vi "Shooter_WinchNoPID.vi"(6 "PickStartPos":dbl, 7 "WinchFiredPos":dbl=3.3, 8 "Winch Pot Location":dbl, 9 "WinchPower":dbl=0.75, 10 "selectedCase":i32, 11 "SetPointArray":dbl[](array[numeric])=[1.0, 2.0, 3.0]) -> (0 "isThere?":bool, 3 "Winch Motor Power Out":dbl)   [LabVIEW 2013]
uses:
  Robot Global Data.vi
panel:
  in  "slow power":dbl=0.45 format="%#_13g"
  out "Winch Desired Location":dbl
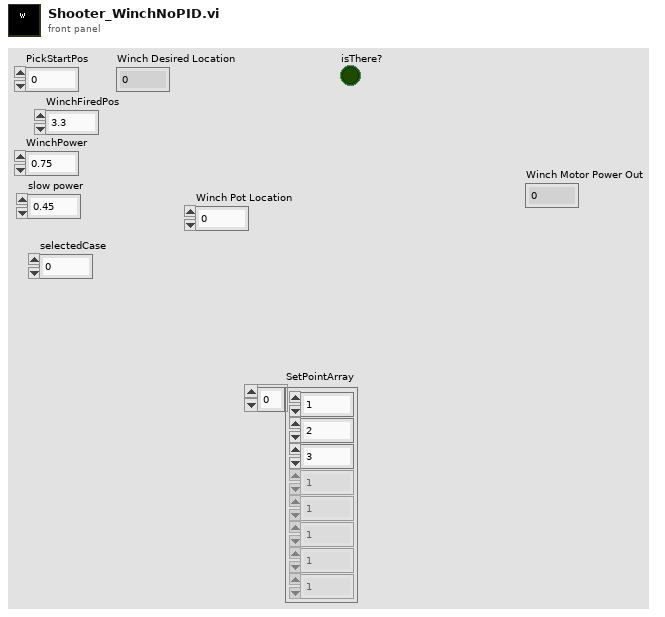
[diagram p1: front panel]
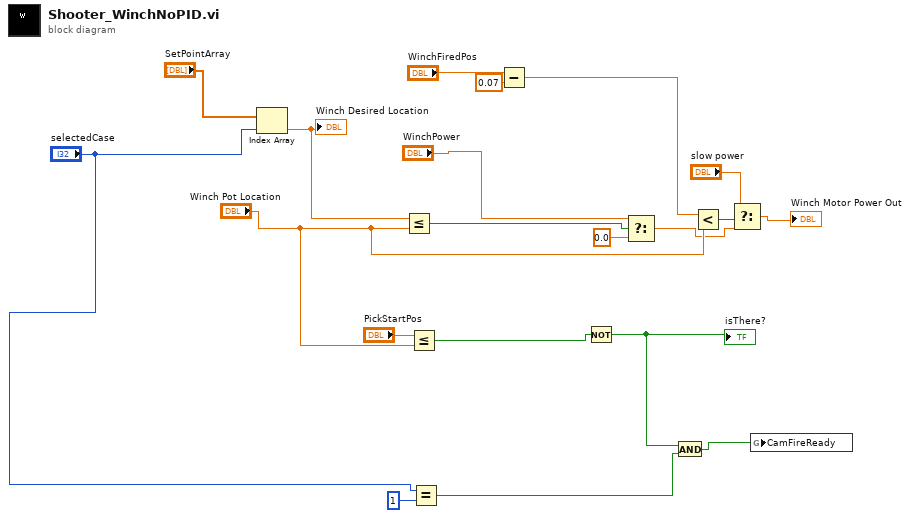
[diagram p0: block diagram]
diagram:
  n1 = Index Array(array="SetPointArray", index="selectedCase") -> (element=w17:dbl)
  "Winch Desired Location" <- w17
  n2 = Less Or Equal?(x=w17, y="Winch Pot Location") -> (x <= y?=w16:bool)
  n3 = Less Or Equal?(x="PickStartPos", y="Winch Pot Location") -> (x <= y?=w15:bool)
  n4 = Equal?(x="selectedCase", y=1) -> (x = y?=w1:bool)
  n5 = Subtract(x="WinchFiredPos", y=0.07) -> (x-y=w7:dbl)
  n6 = Not(x=w15) -> (.not. x?=w5:bool)
  "isThere?" <- w5
  n7 = Select(t="WinchPower", s=w16, f=0.0) -> (s? t:f=w12:dbl)
  n8 = And(x=w5, y=w1) -> (x .and. y?=w4:bool)
  n9 = Less?(x=w7, y="Winch Pot Location") -> (x < y?=w11:bool)
  n10 = Select(t="slow power", s=w11, f=w12) -> (s? t:f=→"Winch Motor Power Out":dbl)
  n11 = global write "Robot Global Data.vi" "CamFireReady"(w4) -> ()
